vi "走合数据.vi"(8 "error in (no error)":errorcluster caption="错误输入（无错误）", 11 "Type":enum16{"Write", "Read"}(ring)) -> (0 "error out":errorcluster caption="错误输出", 3 "file created?":bool)   [LabVIEW 2018]
uses:
  <vilib>/Utility/config.llb/Write Key (String).vi
  <vilib>/Utility/config.llb/Read Key (String).vi
  <vilib>/Utility/config.llb/NI_LVConfig.lvlib
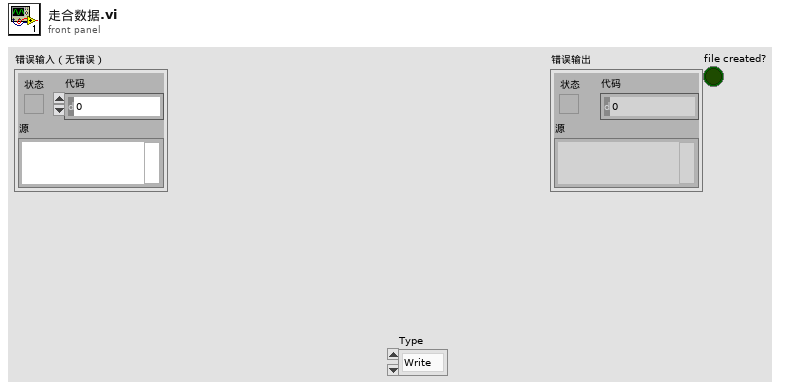
[diagram p1: front panel]
types:
  T1 = typedef "NI_LVConfig.lvlib/Config Data RefNum.ctl" = refnum<k1>
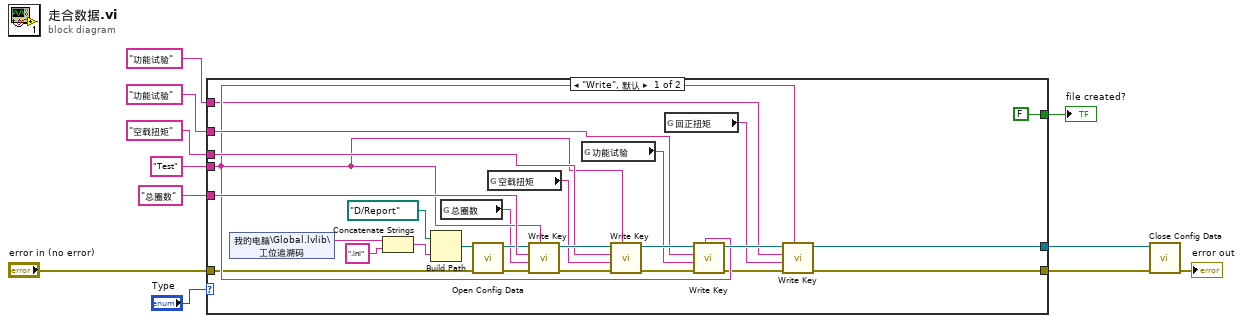
[diagram p0: block diagram]
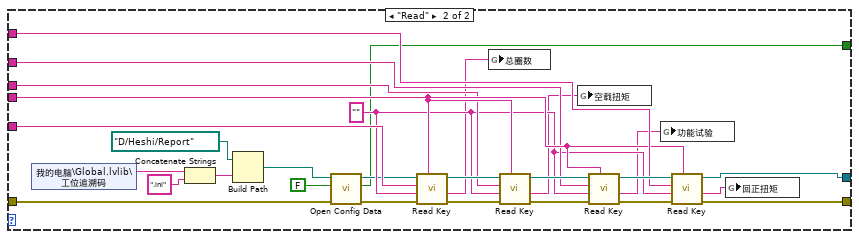
[diagram p2: hidden frame]
diagram:
  n1 = case shown="\"Write\", 默认" "Type" {
    tunnel: "总圈数" ("key") -> [w37 w65]
    tunnel: "空载扭矩" ("key") -> [w35 w58]
    tunnel: "功能试验" ("key") -> [w33 w57]
    tunnel: "Test" ("section") -> [w31 w59]
    tunnel: "功能试验" ("key") -> [w30 w60]
    tunnel: [w29 w61] -> w6
    tunnel: [w25 w52] -> w4
    tunnel: "error in (no error)" -> [w20 w51]
    tunnel: [FALSE ("file created?") w38] -> w1
    frame "Write", Default {
      n2 = shared-variable "我的电脑\\Global.lvlib\\工位追溯码"() -> (w23:string)  [unwired: 1 in, 1 out]
      n3 = Concatenate Strings(w23, ".ini" ("字符串")) -> (w24:string)
      n4 = Build Path(base path=path "D:/Report" ("文件路径（使用对话框）"), name or relative path=w24) -> (appended path=w21:path)
      n5 = global read "检测结果.vi" "总圈数"() -> (w16:string)
      n6 = call <vilib>:"Open Config Data.vi"("error in (no error)"=w20, "configuration file path"=w21) -> ("error out"=w19:errorcluster, "refnum"=w18:T1)  [unwired: 7 in, 1 out]
      n7 = global read "检测结果.vi" "空载扭矩"() -> (w15:string)
      n8 = call-poly <vilib>:"Write Key.vi"("section"=w31, "error in (no error)"=w19, "value"=w16, "key"=w37, "refnum"=w18) -> ("error out"=w28:errorcluster, "refnum out"=w36:T1)  [unwired: 4 in, 1 out]
      n9 = global read "检测结果.vi" "功能试验"() -> (w14:string)
      n10 = call-poly <vilib>:"Write Key.vi"("section"=w31, "error in (no error)"=w28, "value"=w15, "key"=w35, "refnum"=w36) -> ("error out"=w27:errorcluster, "refnum out"=w34:T1)  [unwired: 4 in, 1 out]
      n11 = global read "检测结果.vi" "回正扭矩"() -> (w13:string)
      n12 = call-poly <vilib>:"Write Key.vi"("section"=w31, "error in (no error)"=w27, "value"=w14, "key"=w33, "refnum"=w34) -> ("error out"=w26:errorcluster, "refnum out"=w32:T1)  [unwired: 4 in, 1 out]
      n13 = call-poly <vilib>:"Write Key.vi"("section"=w31, "error in (no error)"=w26, "value"=w13, "key"=w30, "refnum"=w32) -> ("error out"=w25:errorcluster, "refnum out"=w29:T1)  [unwired: 4 in, 1 out]
    }
    frame "Read" {
      w56 = "" ("default value")
      n14 = shared-variable "我的电脑\\Global.lvlib\\工位追溯码"() -> (w47:string)  [unwired: 1 in, 1 out]
      n15 = Concatenate Strings(w47, ".ini" ("字符串")) -> (w48:string)
      n16 = Build Path(base path=path "D:/Heshi/Report" ("文件路径（使用对话框）"), name or relative path=w48) -> (appended path=w44:path)
      n17 = call <vilib>:"Open Config Data.vi"("error in (no error)"=w51, "create file if necessary (T)"=FALSE, "configuration file path"=w44) -> ("error out"=w50:errorcluster, "file created?"=w38:bool, "refnum"=w49:T1)  [unwired: 6 in]
      n18 = call-poly <vilib>:"Read Key.vi"("section"=w59, "error in (no error)"=w50, "default value"=w56, "key"=w65, "refnum"=w49) -> ("error out"=w55:errorcluster, "value"=w40:string, "refnum out"=w64:T1)  [unwired: 3 in, 1 out]
      n19 = global write "检测结果.vi" "总圈数"(w40) -> ()
      n20 = call-poly <vilib>:"Read Key.vi"("section"=w59, "error in (no error)"=w55, "default value"=w56, "key"=w58, "refnum"=w64) -> ("error out"=w54:errorcluster, "value"=w41:string, "refnum out"=w63:T1)  [unwired: 3 in, 1 out]
      n21 = global write "检测结果.vi" "空载扭矩"(w41) -> ()
      n22 = call-poly <vilib>:"Read Key.vi"("section"=w59, "error in (no error)"=w54, "default value"=w56, "key"=w57, "refnum"=w63) -> ("error out"=w53:errorcluster, "value"=w42:string, "refnum out"=w62:T1)  [unwired: 3 in, 1 out]
      n23 = global write "检测结果.vi" "功能试验"(w42) -> ()
      n24 = call-poly <vilib>:"Read Key.vi"("section"=w59, "error in (no error)"=w53, "default value"=w56, "key"=w60, "refnum"=w62) -> ("error out"=w52:errorcluster, "value"=w43:string, "refnum out"=w61:T1)  [unwired: 3 in, 1 out]
      n25 = global write "检测结果.vi" "回正扭矩"(w43) -> ()
    }
  }
  "file created?" <- w1
  n26 = call <vilib>:"Close Config Data.vi"("error in (no error)"=w4, "refnum"=w6) -> ("error out"=→"error out":errorcluster)  [unwired: 8 in, 1 out]
